vi "joystick scaleNtransform.vi"(9 "joystick values":dbl[](array[numeric])) -> (3 "Transformed joystick values":dbl[](array[numeric]))   [LabVIEW 2019]
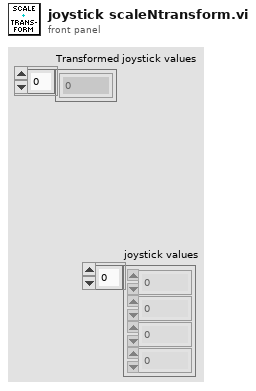
[diagram p1: front panel]
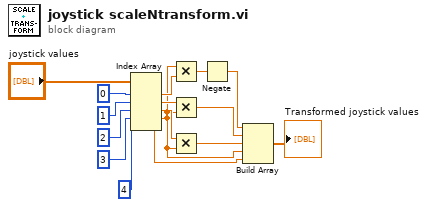
[diagram p0: block diagram]
diagram:
  n1 = Index Array(array="joystick values", index #1=0 ("index"), index #2=1 ("index"), index #3=2 ("index"), index #4=3 ("index"), index #5=4 ("index")) -> (element #1=w11:dbl, element #2=w10:dbl, element #3=w9:dbl, element #4=w3:dbl, element #5=w2:dbl)
  n2 = Multiply(x=w3, y=w11) -> (x*y=w8:dbl)
  n3 = Multiply(x=w10, y=w3) -> (x*y=w6:dbl)
  n4 = Multiply(x=w9, y=w3) -> (x*y=w4:dbl)
  n5 = Negate(x=w8) -> (-x=w7:dbl)
  n6 = Build Array(w7, w6, w4, w3, w2) -> (→"Transformed joystick values":dbl[])
